vi "Add To.vi"(8 "error in (no error)":errorcluster, 10 "To":T1, 11 "Gmail in":refnum<class "Gmail.lvclass">) -> (0 "error out":errorcluster, 3 "Gmail out":refnum<class "Gmail.lvclass">)   [LabVIEW 2020, in "Gmail API.lvlib" / "Gmail.lvclass"]
uses:
  Gmail.lvclass
  Mail Address.ctl
  Gmail.lvclass/Gmail.ctl
  Gmail API.lvlib
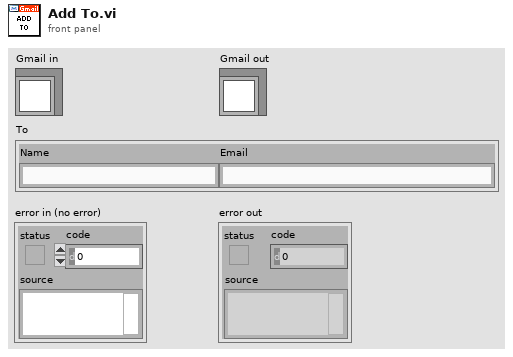
[diagram p1: front panel]
types:
  T1 = typedef "Gmail API.lvlib/Mail Address.ctl" = cluster{"Name":string, "Email":string}
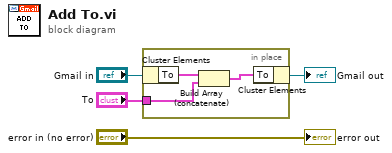
[diagram p0: block diagram]
diagram:
  n1 = in-place {
    in-place-border: "To" -> [w5]
    n2 = in-place-cluster #1("Gmail in") -> ("To"=w7:T1[])
    n3 = Build Array (concatenate)(w7, w5) -> (w6:T1[])
    n4 = in-place-cluster #1("To"=w6) -> (→"Gmail out":refnum<class "Gmail.lvclass">)
  }
  "error out" <- "error in (no error)"
